vi "System_Host.vi"() -> ()   [LabVIEW 2017]
uses:
  <vilib>/Analysis/baseanly.llb/Mean (DBL).vi
  <vilib>/Utility/file.llb/Read Delimited Spreadsheet (string).vi
  <vilib>/Utility/file.llb/Write Delimited Spreadsheet (string).vi
  <vilib>/Utility/file.llb/Read Delimited Spreadsheet (DBL).vi
  <vilib>/Utility/file.llb/Write Delimited Spreadsheet (DBL).vi
  <resource>/objmgr/ni.dex.rc
  <vilib>/Analysis/NI_AALBase.lvlib
panel:
  in  "Flow Data?":bool=TRUE
  out "System Safe":bool
  in  "Exit Profile":bool
  in  "Select Operation Mode":T1(ring) caption="Select Operation Mode2"
  in  "CTAH Frequency\n[10*Hz]":u16
  out "System Time [s]":sgl
  out "System Loop Time (ms)":u32
  in  "Load Power Profile":bool
  in  "Dyn. Power Profile File":path
  out "CTAH Temperatures":T2(graph)
  out "CTAH Outlet":dbl format="%0.2f"
  out "CTAH Inlet":dbl format="%0.2f"
  out "Core Temperatures":T2(graph)
  out "Heater Outlet":dbl format="%0.2f"
  out "Heater Inlet":dbl format="%0.2f"
  out "Core Power":T2(graph)
  out "FM-60 [kg/s]":sgl
  out "FM-40 [kg/s]":sgl
  out "FM-30 [kg/s]":sgl
  out "FM-20 [kg/s]":sgl
  in  "Tab Control":enum32{"Thermocouple Readings [C]"}(tab)
  out "WT-10":sgl
  out "BT-11":sgl
  out "BT-12":sgl
  out "WT-13":sgl
  out "CX-10":dbl format="%0.2f"
  out "CX-11":dbl format="%0.2f"
  out "WT-20":sgl
  out "BT-21":sgl
  out "WT-22":sgl
  out "BT-23":sgl
  out "WT-24":sgl
  out "BT-25":sgl
  out "WT-26":sgl
  out "BT-27":sgl
  out "WT-28":sgl
  out "BT-29":sgl
  out "BT-30":sgl
  out "WT-31":sgl
  out "BT-32":sgl
  out "WT-33":sgl
  out "BT-34":sgl
  out "WT-35":sgl
  out "WT-40":sgl
  out "BT-41":sgl
  out "WT-42":sgl
  out "BT-43":sgl
  out "BT-60":sgl
  out "WT-61":sgl
  out "WT-62":sgl
  out "BT-63":sgl
  out "WT-64":sgl
  out "BT-65":sgl
  out "BT-66":sgl
  out "WT-67":sgl
  out "ST-10":sgl
  out "ST-11":sgl
  out "ST-12":sgl[](array[numeric])
  out "ST-13":sgl
  out "ST-14":sgl[](array[numeric])
  out "AT-01":sgl
  out "AT-02":sgl
  out "Profile Step":i32
  out "Power Output [W]":dbl
  out "Power Input Signal [W]":dbl
  out "Output Current 2 [A]":dbl
  out "Output Voltage 2 [V]":dbl
  out "Output Current 1 [A]":dbl
  out "Output Voltage 1 [V]":dbl
  out "Loop Period [ms]":i64
  in  "Shutdown":bool
  in  "Desired Power [W]":dbl
  in  "Power Output On":bool
  in  "Pump Frequency\n[10*Hz]":u16
  in  "ACTIVATE - PUMP":bool
  in  "Pump Operation Mode":i32(listbox)
  in  "TCHX Frequency\n[10*Hz]":u16
  in  "ACTIVATE - TCHX":bool
  in  "TCHX Operation Mode":i32(listbox)
  in  "VFD Stop":bool
  in  "ACTIVATE - CTAH":bool
  in  "CTAH Operation Mode":i32(listbox)
  in  "Error In":errorcluster
  out "Number of Disconnections":u32
  out "Available Elements for Reading":i32
  out "DAQ?":bool
  in  "Stop DAQ":bool
  out "Error Out":errorcluster
  # ".csv file with single column\nAssume constant loop frequency (1 Hz)"
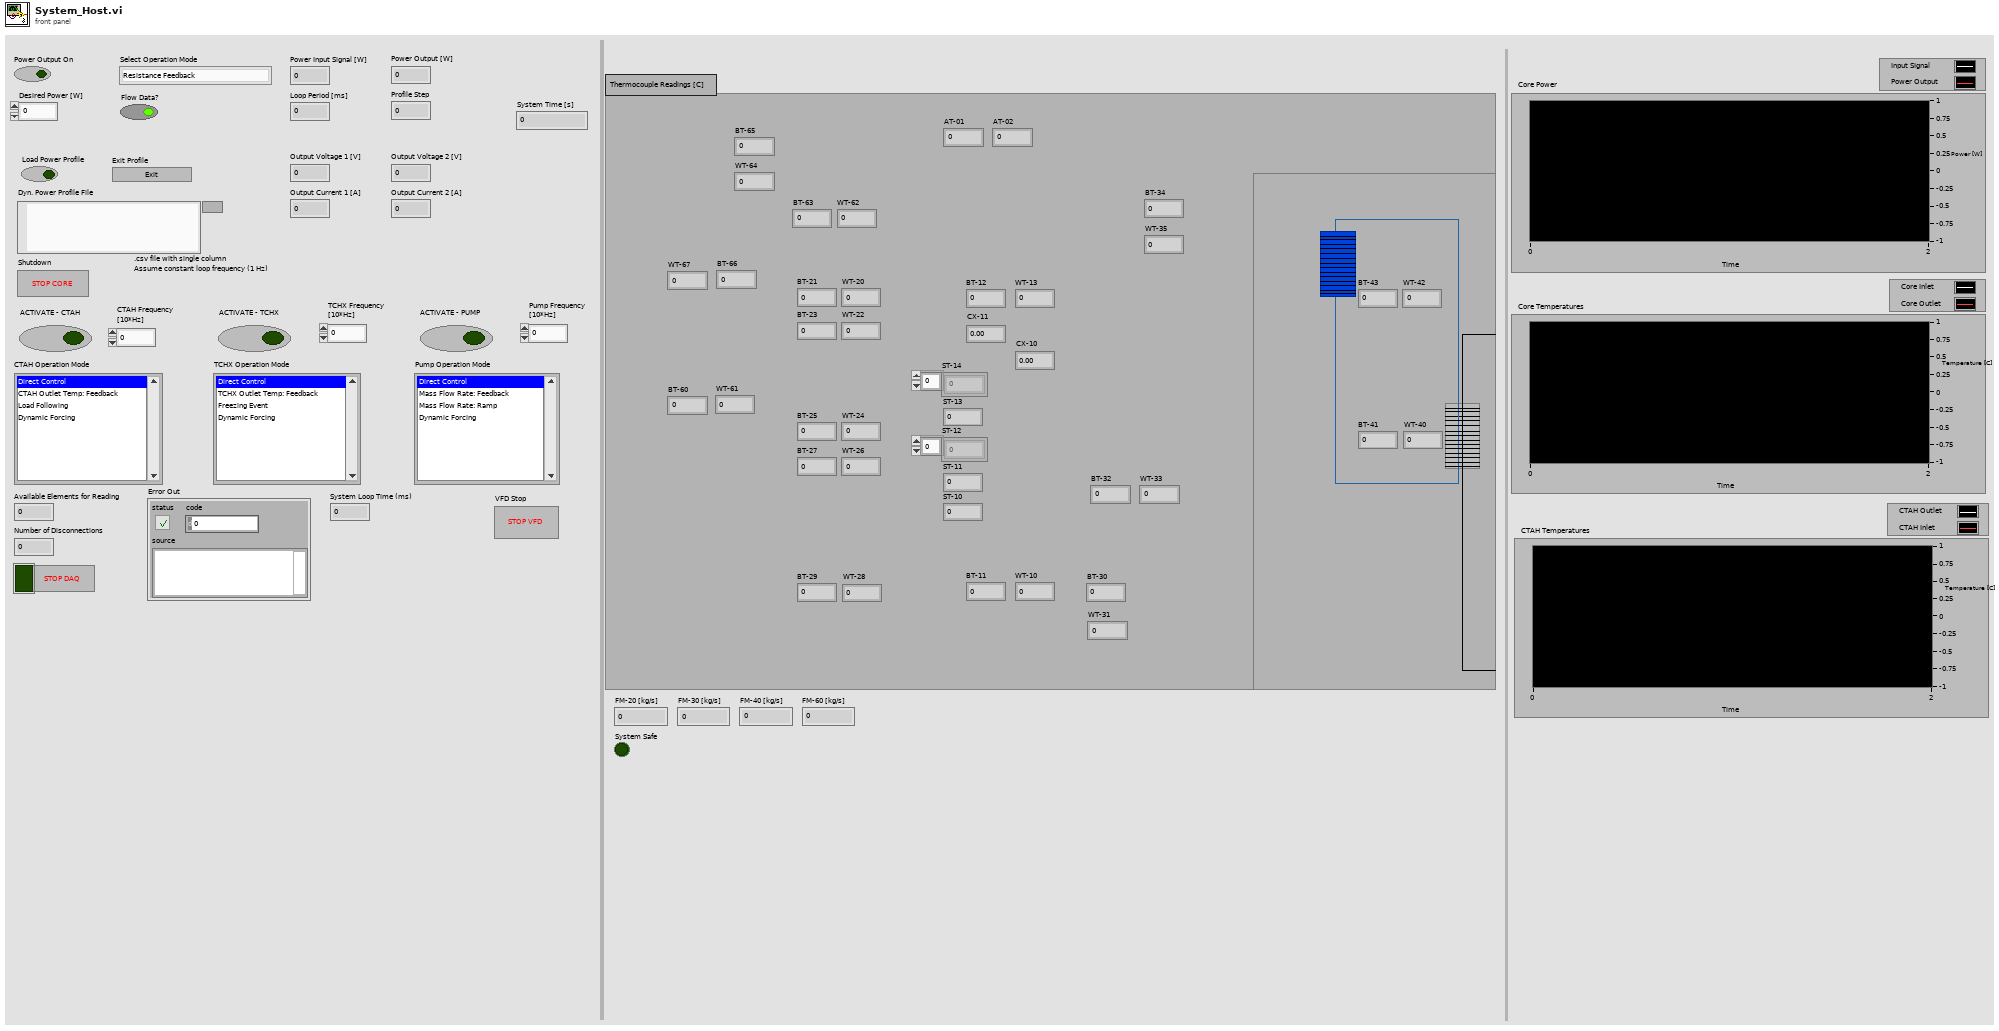
[diagram p1: front panel]
types:
  T1 = enum16{"Resistance Feedback", "Power Profile Input", "Resistance Feedback_Analog", "Power Profile Input_Analog", "SNF Digital", "SNF Analog\n", "Shutdown"}
  T2 = cluster{"Power Input Signal":dbl, "Power Output":dbl}
  T3 = cluster{"Power Input Signal [W]":dbl, "Power Output [W]":dbl}
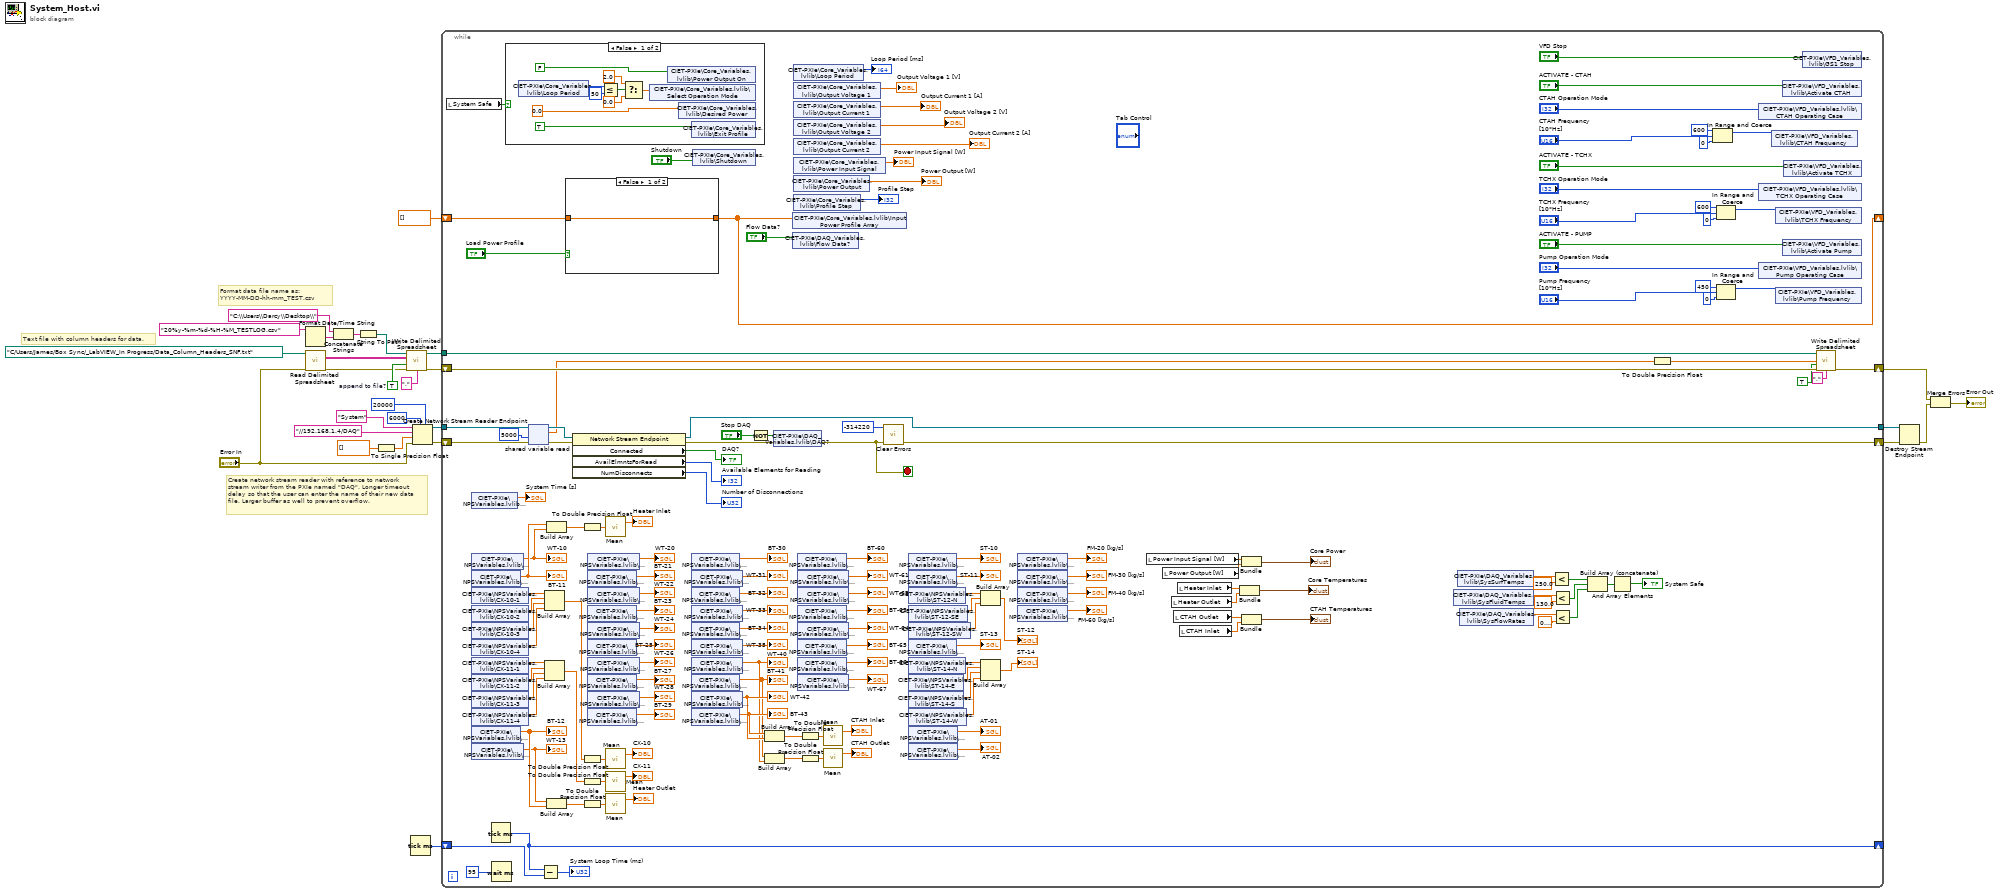
[diagram p0: block diagram]
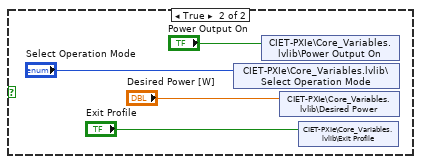
[diagram p2: hidden frame]
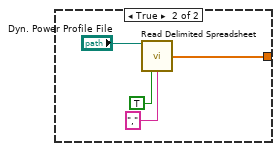
[diagram p3: hidden frame]
diagram:
  w15 = TRUE  # append to file?
  # "Format data file name as:\nYYYY-MM-DD-hh-mm_TEST.csv"
  # "Create network stream reader with reference to network\nstream writer from the PXIe named \"DAQ\". Longer timeout\ndelay so that the user can enter the name of their new data\nfile. Larger buffer as well to prevent overflow."
  # "Text file with column headers for data."
  n1 = Format Date/Time String(time format string (%c)="20%y-%m-%d-%H-%M_TESTLOG.csv") -> (date/time string=w5:string)  [unwired: 2 in]
  n2 = call-poly <vilib>:"Read Delimited Spreadsheet.vi"("file path (dialog if empty)"=path "C:/Users/James/Box Sync/_LabVIEW_In Progress/Data_Column_Headers_SNF.txt", "error in (no error)"="Error In") -> ("all rows"=w18:string[][], "error out"=w13:errorcluster)  [unwired: 8 in, 4 out]
  n3 = Concatenate Strings("C:\\Users\\Darcy\\Desktop\\" ("string"), w5) -> (w7:string)
  n4 = String To Path(string=w7) -> (path=w4:path)
  n5 = To Single Precision Float(number=dbl[] []) -> (single precision float=w26:sgl[])
  n6 = call-poly <vilib>:"Write Delimited Spreadsheet.vi"("file path (dialog if empty)"=w4, "2D data"=w18, "append to file? (new file:F)"=w15, "error in (no error)"=w13, "delimiter (\\t)"=",") -> ("new file path (Not A Path if cancelled)"=w14:path, "error out"=w12:errorcluster)  [unwired: 9 in]
  n7 = Tick Count (ms)() -> (millisecond timer value=w1:u32)
  n8 = Create Network Stream Reader Endpoint(5:20000 ("timeout in ms (-1)"), 7:6000 ("reader buffer size"), 8:"Error In", 9:w26, 10:"//192.168.1.4/DAQ" ("writer url"), 11:"System" ("reader name")) -> (0:w23:errorcluster, 3:w22:refnum<k21>)  [unwired: 1 in]
  n9 = while {
    shift-right: [w173] -> w21
    shift-left: w23 -> [w181]
    tunnel: w22 -> [w182]
    tunnel: [w172] -> w20
    tunnel: w14 -> [w168]
    shift-right: [w166] -> w11
    shift-left: w12 -> [w167]
    shift-right: [w52] -> _
    shift-left: dbl[] [] ("Input Power Profile Array") -> [w53]
    shift-right: [w49] -> _
    shift-left: w1 -> [w50]
    stop <- w171 stop-if-true
    n10 = local read "System Safe"() -> (w31:bool)
    n11 = shared-variable "CIET-PXIe\\NPSVariables.lvlib\\Time"() -> (→"System Time [s]":sgl)  [unwired: 1 in, 1 out]
    n12 = shared-variable "CIET-PXIe\\NPSVariables.lvlib\\WT-10"() -> (w73:sgl)  [unwired: 1 in, 1 out]
    "WT-10" <- w73
    n13 = shared-variable "CIET-PXIe\\NPSVariables.lvlib\\BT-11"() -> (w74:sgl)  [unwired: 1 in, 1 out]
    "BT-11" <- w74
    n14 = shared-variable "CIET-PXIe\\NPSVariables.lvlib\\CX-10-1"() -> (w139:sgl)  [unwired: 1 in, 1 out]
    n15 = shared-variable "CIET-PXIe\\NPSVariables.lvlib\\CX-10-2"() -> (w138:sgl)  [unwired: 1 in, 1 out]
    n16 = shared-variable "CIET-PXIe\\NPSVariables.lvlib\\CX-10-3"() -> (w137:sgl)  [unwired: 1 in, 1 out]
    n17 = shared-variable "CIET-PXIe\\NPSVariables.lvlib\\CX-10-4"() -> (w136:sgl)  [unwired: 1 in, 1 out]
    n18 = shared-variable "CIET-PXIe\\NPSVariables.lvlib\\CX-11-1"() -> (w132:sgl)  [unwired: 1 in, 1 out]
    n19 = shared-variable "CIET-PXIe\\NPSVariables.lvlib\\CX-11-2"() -> (w131:sgl)  [unwired: 1 in, 1 out]
    n20 = shared-variable "CIET-PXIe\\NPSVariables.lvlib\\CX-11-3"() -> (w130:sgl)  [unwired: 1 in, 1 out]
    n21 = shared-variable "CIET-PXIe\\NPSVariables.lvlib\\CX-11-4"() -> (w129:sgl)  [unwired: 1 in, 1 out]
    n22 = shared-variable "CIET-PXIe\\NPSVariables.lvlib\\BT-12"() -> (w78:sgl)  [unwired: 1 in, 1 out]
    "BT-12" <- w78
    n23 = shared-variable "CIET-PXIe\\NPSVariables.lvlib\\WT-13"() -> (w77:sgl)  [unwired: 1 in, 1 out]
    "WT-13" <- w77
    n24 = Tick Count (ms)() -> (millisecond timer value=w49:u32)
    n25 = Wait (ms)(milliseconds to wait=u32 95) -> ()  [unwired: 1 out]
    n26 = case shown="False" w31 {
      frame False {
        n27 = shared-variable "CIET-PXIe\\Core_Variables.lvlib\\Loop Period"() -> (w189:i64)  [unwired: 1 in, 1 out]
        n28 = Less Or Equal?(x=w189, y=i64 50) -> (x <= y?=w190:bool)
        n29 = Select(t=2.0, s=w190, f=0.0) -> (s? t:f=w185:dbl)
        n30 = shared-variable "CIET-PXIe\\Core_Variables.lvlib\\Select Operation Mode"(w185) -> ()  [unwired: 1 in, 1 out]
        n31 = shared-variable "CIET-PXIe\\Core_Variables.lvlib\\Power Output On"(FALSE ("Power Output On")) -> ()  [unwired: 1 in, 1 out]
        n32 = shared-variable "CIET-PXIe\\Core_Variables.lvlib\\Desired Power"(0.0 ("Desired Power")) -> ()  [unwired: 1 in, 1 out]
        n33 = shared-variable "CIET-PXIe\\Core_Variables.lvlib\\Exit Profile"(TRUE ("Exit Profile")) -> ()  [unwired: 1 in, 1 out]
      }
      frame True {
        n34 = shared-variable "CIET-PXIe\\Core_Variables.lvlib\\Select Operation Mode"("Select Operation Mode") -> ()  [unwired: 1 in, 1 out]
        n35 = shared-variable "CIET-PXIe\\Core_Variables.lvlib\\Power Output On"("Power Output On") -> ()  [unwired: 1 in, 1 out]
        n36 = shared-variable "CIET-PXIe\\Core_Variables.lvlib\\Desired Power"("Desired Power [W]") -> ()  [unwired: 1 in, 1 out]
        n37 = shared-variable "CIET-PXIe\\Core_Variables.lvlib\\Exit Profile"("Exit Profile") -> ()  [unwired: 1 in, 1 out]
      }
    }
    n38 = shared-variable-read(w182, w181, 5000 ("timeout ms (-1)")) -> (w178:refnum<k21>, w176:errorcluster, w140:sgl[])  [unwired: 1 out]
    n39 = Subtract(x=w49, y=w50) -> (x-y=→"System Loop Time (ms)":u32)
    n40 = Build Array(w139, w138, w137, w136) -> (w135:sgl[])
    n41 = Build Array(w132, w131, w130, w129) -> (w128:sgl[])
    n42 = Build Array(w74, w73) -> (w75:sgl[])
    n43 = Build Array(w77, w78) -> (w79:sgl[])
    n44 = case shown="False" "Load Power Profile" {
      tunnel: [w198 w199] -> w52
      tunnel: w53 -> [w198 _]
      frame False {
      }
      frame True {
        n45 = call-poly <vilib>:"Read Delimited Spreadsheet.vi"("file path (dialog if empty)"="Dyn. Power Profile File", "transpose? (F)"=TRUE, "delimiter (\\t)"="," ("delimiter (\\t)")) -> ("first row"=w199:dbl[])  [unwired: 7 in, 5 out]
      }
    }
    n46 = property class="Network Stream Endpoint"(reference=w178, error in=w176) -> (reference out=w172:refnum<k21>, error out=w177:errorcluster, "Connected"=→"DAQ?":bool, "AvailElmntsForRead"=→"Available Elements for Reading":i32, "NumDisconnects"=→"Number of Disconnections":u32)
    n47 = To Double Precision Float(number=w75) -> (double precision float=w76:dbl[])
    n48 = To Double Precision Float(number=w135) -> (double precision float=w134:dbl[])
    n49 = To Double Precision Float(number=w128) -> (double precision float=w133:dbl[])
    n50 = To Double Precision Float(number=w79) -> (double precision float=w80:dbl[])
    n51 = shared-variable "CIET-PXIe\\NPSVariables.lvlib\\WT-20"() -> (→"WT-20":sgl)  [unwired: 1 in, 1 out]
    n52 = shared-variable "CIET-PXIe\\NPSVariables.lvlib\\BT-21"() -> (→"BT-21":sgl)  [unwired: 1 in, 1 out]
    n53 = shared-variable "CIET-PXIe\\NPSVariables.lvlib\\WT-22"() -> (→"WT-22":sgl)  [unwired: 1 in, 1 out]
    n54 = shared-variable "CIET-PXIe\\NPSVariables.lvlib\\BT-23"() -> (→"BT-23":sgl)  [unwired: 1 in, 1 out]
    n55 = shared-variable "CIET-PXIe\\NPSVariables.lvlib\\WT-24"() -> (→"WT-24":sgl)  [unwired: 1 in, 1 out]
    n56 = shared-variable "CIET-PXIe\\NPSVariables.lvlib\\BT-25"() -> (→"BT-25":sgl)  [unwired: 1 in, 1 out]
    n57 = shared-variable "CIET-PXIe\\NPSVariables.lvlib\\WT-26"() -> (→"WT-26":sgl)  [unwired: 1 in, 1 out]
    n58 = shared-variable "CIET-PXIe\\NPSVariables.lvlib\\BT-27"() -> (→"BT-27":sgl)  [unwired: 1 in, 1 out]
    n59 = shared-variable "CIET-PXIe\\NPSVariables.lvlib\\WT-28"() -> (→"WT-28":sgl)  [unwired: 1 in, 1 out]
    n60 = shared-variable "CIET-PXIe\\NPSVariables.lvlib\\BT-29"() -> (→"BT-29":sgl)  [unwired: 1 in, 1 out]
    n61 = call-poly <vilib>:"Mean.vi"("X"=w76) -> ("mean"=→"Heater Inlet":dbl)  [unwired: 1 out]
    n62 = call-poly <vilib>:"Mean.vi"("X"=w134) -> ("mean"=→"CX-10":dbl)  [unwired: 1 out]
    n63 = call-poly <vilib>:"Mean.vi"("X"=w133) -> ("mean"=→"CX-11":dbl)  [unwired: 1 out]
    n64 = call-poly <vilib>:"Mean.vi"("X"=w80) -> ("mean"=→"Heater Outlet":dbl)  [unwired: 1 out]
    n65 = shared-variable "CIET-PXIe\\NPSVariables.lvlib\\BT-30"() -> (→"BT-30":sgl)  [unwired: 1 in, 1 out]
    n66 = shared-variable "CIET-PXIe\\NPSVariables.lvlib\\WT-31"() -> (→"WT-31":sgl)  [unwired: 1 in, 1 out]
    n67 = shared-variable "CIET-PXIe\\NPSVariables.lvlib\\BT-32"() -> (→"BT-32":sgl)  [unwired: 1 in, 1 out]
    n68 = shared-variable "CIET-PXIe\\NPSVariables.lvlib\\WT-33"() -> (→"WT-33":sgl)  [unwired: 1 in, 1 out]
    n69 = shared-variable "CIET-PXIe\\NPSVariables.lvlib\\BT-34"() -> (→"BT-34":sgl)  [unwired: 1 in, 1 out]
    n70 = shared-variable "CIET-PXIe\\NPSVariables.lvlib\\WT-35"() -> (→"WT-35":sgl)  [unwired: 1 in, 1 out]
    n71 = shared-variable "CIET-PXIe\\NPSVariables.lvlib\\WT-40"() -> (w59:sgl)  [unwired: 1 in, 1 out]
    "WT-40" <- w59
    n72 = shared-variable "CIET-PXIe\\NPSVariables.lvlib\\BT-41"() -> (w58:sgl)  [unwired: 1 in, 1 out]
    "BT-41" <- w58
    n73 = shared-variable "CIET-PXIe\\NPSVariables.lvlib\\WT-42"() -> (w61:sgl)  [unwired: 1 in, 1 out]
    "WT-42" <- w61
    n74 = shared-variable "CIET-PXIe\\NPSVariables.lvlib\\BT-43"() -> (w60:sgl)  [unwired: 1 in, 1 out]
    "BT-43" <- w60
    n75 = shared-variable "CIET-PXIe\\Core_Variables.lvlib\\Shutdown"("Shutdown") -> ()  [unwired: 1 in, 1 out]
    n76 = Not(x="Stop DAQ") -> (.not. x?=w180:bool)
    n77 = Build Array(w60, w61) -> (w66:sgl[])
    n78 = Build Array(w58, w59) -> (w63:sgl[])
    n79 = shared-variable "CIET-PXIe\\DAQ_Variables.lvlib\\DAQ?"(w180, error in=w177) -> (error out=w171:errorcluster)
    n80 = shared-variable "CIET-PXIe\\Core_Variables.lvlib\\Input Power Profile Array"(w52) -> ()  [unwired: 1 in, 1 out]
    n81 = shared-variable "CIET-PXIe\\DAQ_Variables.lvlib\\Flow Data?"("Flow Data?") -> ()  [unwired: 1 in, 1 out]
    n82 = shared-variable "CIET-PXIe\\Core_Variables.lvlib\\Loop Period"() -> (→"Loop Period [ms]":i64)  [unwired: 1 in, 1 out]
    n83 = shared-variable "CIET-PXIe\\Core_Variables.lvlib\\Output Voltage 1"() -> (→"Output Voltage 1 [V]":dbl)  [unwired: 1 in, 1 out]
    n84 = shared-variable "CIET-PXIe\\Core_Variables.lvlib\\Output Current 1"() -> (→"Output Current 1 [A]":dbl)  [unwired: 1 in, 1 out]
    n85 = shared-variable "CIET-PXIe\\Core_Variables.lvlib\\Output Voltage 2"() -> (→"Output Voltage 2 [V]":dbl)  [unwired: 1 in, 1 out]
    n86 = shared-variable "CIET-PXIe\\Core_Variables.lvlib\\Output Current 2"() -> (→"Output Current 2 [A]":dbl)  [unwired: 1 in, 1 out]
    n87 = shared-variable "CIET-PXIe\\Core_Variables.lvlib\\Power Input Signal"() -> (→"Power Input Signal [W]":dbl)  [unwired: 1 in, 1 out]
    n88 = shared-variable "CIET-PXIe\\Core_Variables.lvlib\\Power Output"() -> (→"Power Output [W]":dbl)  [unwired: 1 in, 1 out]
    n89 = shared-variable "CIET-PXIe\\Core_Variables.lvlib\\Profile Step"() -> (→"Profile Step":i32)  [unwired: 1 in, 1 out]
    n90 = shared-variable "CIET-PXIe\\NPSVariables.lvlib\\BT-60"() -> (→"BT-60":sgl)  [unwired: 1 in, 1 out]
    n91 = shared-variable "CIET-PXIe\\NPSVariables.lvlib\\WT-61"() -> (→"WT-61":sgl)  [unwired: 1 in, 1 out]
    n92 = shared-variable "CIET-PXIe\\NPSVariables.lvlib\\WT-62"() -> (→"WT-62":sgl)  [unwired: 1 in, 1 out]
    n93 = shared-variable "CIET-PXIe\\NPSVariables.lvlib\\BT-63"() -> (→"BT-63":sgl)  [unwired: 1 in, 1 out]
    n94 = shared-variable "CIET-PXIe\\NPSVariables.lvlib\\WT-64"() -> (→"WT-64":sgl)  [unwired: 1 in, 1 out]
    n95 = shared-variable "CIET-PXIe\\NPSVariables.lvlib\\BT-65"() -> (→"BT-65":sgl)  [unwired: 1 in, 1 out]
    n96 = shared-variable "CIET-PXIe\\NPSVariables.lvlib\\BT-66"() -> (→"BT-66":sgl)  [unwired: 1 in, 1 out]
    n97 = shared-variable "CIET-PXIe\\NPSVariables.lvlib\\WT-67"() -> (→"WT-67":sgl)  [unwired: 1 in, 1 out]
    n98 = To Double Precision Float(number=w66) -> (double precision float=w67:dbl[])
    n99 = To Double Precision Float(number=w63) -> (double precision float=w64:dbl[])
    n100 = call-poly <vilib>:"Mean.vi"("X"=w67) -> ("mean"=→"CTAH Inlet":dbl)  [unwired: 1 out]
    n101 = call-poly <vilib>:"Mean.vi"("X"=w64) -> ("mean"=→"CTAH Outlet":dbl)  [unwired: 1 out]
    n102 = call <vilib>:"Clear Errors.vi"("error in (no error)"=w171, "specific error code to clear (0: all)"=-314220) -> ("error out"=w173:errorcluster)  [unwired: 4 in, 1 out]
    n103 = shared-variable "CIET-PXIe\\NPSVariables.lvlib\\ST-10"() -> (→"ST-10":sgl)  [unwired: 1 in, 1 out]
    n104 = shared-variable "CIET-PXIe\\NPSVariables.lvlib\\ST-11"() -> (→"ST-11":sgl)  [unwired: 1 in, 1 out]
    n105 = shared-variable "CIET-PXIe\\NPSVariables.lvlib\\ST-12-N"() -> (w99:sgl)  [unwired: 1 in, 1 out]
    n106 = shared-variable "CIET-PXIe\\NPSVariables.lvlib\\ST-12-SE"() -> (w98:sgl)  [unwired: 1 in, 1 out]
    n107 = shared-variable "CIET-PXIe\\NPSVariables.lvlib\\ST-12-SW"() -> (w97:sgl)  [unwired: 1 in, 1 out]
    n108 = shared-variable "CIET-PXIe\\NPSVariables.lvlib\\ST-13"() -> (→"ST-13":sgl)  [unwired: 1 in, 1 out]
    n109 = shared-variable "CIET-PXIe\\NPSVariables.lvlib\\ST-14-N"() -> (w94:sgl)  [unwired: 1 in, 1 out]
    n110 = shared-variable "CIET-PXIe\\NPSVariables.lvlib\\ST-14-E"() -> (w93:sgl)  [unwired: 1 in, 1 out]
    n111 = shared-variable "CIET-PXIe\\NPSVariables.lvlib\\ST-14-S"() -> (w92:sgl)  [unwired: 1 in, 1 out]
    n112 = shared-variable "CIET-PXIe\\NPSVariables.lvlib\\ST-14-W"() -> (w91:sgl)  [unwired: 1 in, 1 out]
    n113 = shared-variable "CIET-PXIe\\NPSVariables.lvlib\\AT-01"() -> (→"AT-01":sgl)  [unwired: 1 in, 1 out]
    n114 = shared-variable "CIET-PXIe\\NPSVariables.lvlib\\AT-02"() -> (→"AT-02":sgl)  [unwired: 1 in, 1 out]
    n115 = Build Array(w99, w98, w97) -> (→"ST-12":sgl[])
    n116 = Build Array(w94, w93, w92, w91) -> (→"ST-14":sgl[])
    n117 = shared-variable "CIET-PXIe\\NPSVariables.lvlib\\FM-20"() -> (→"FM-20 [kg/s]":sgl)  [unwired: 1 in, 1 out]
    n118 = shared-variable "CIET-PXIe\\NPSVariables.lvlib\\FM-30"() -> (→"FM-30 [kg/s]":sgl)  [unwired: 1 in, 1 out]
    n119 = shared-variable "CIET-PXIe\\NPSVariables.lvlib\\FM-40"() -> (→"FM-40 [kg/s]":sgl)  [unwired: 1 in, 1 out]
    n120 = shared-variable "CIET-PXIe\\NPSVariables.lvlib\\FM-60"() -> (→"FM-60 [kg/s]":sgl)  [unwired: 1 in, 1 out]
    n121 = local read "Power Input Signal [W]"() -> (w83:dbl)
    n122 = local read "Power Output [W]"() -> (w82:dbl)
    n123 = local read "Heater Outlet"() -> (w68:dbl)
    n124 = local read "CTAH Outlet"() -> (w56:dbl)
    n125 = local read "Heater Inlet"() -> (w69:dbl)
    n126 = local read "CTAH Inlet"() -> (w55:dbl)
    n127 = Bundle("Heater Inlet"=w69, "Heater Outlet"=w68) -> (→"Core Temperatures":cluster{"Heater Inlet":dbl, "Heater Outlet":dbl})  [unwired: 1 in]
    n128 = Bundle("Power Input Signal [W]"=w83, "Power Output [W]"=w82) -> (→"Core Power":T3)  [unwired: 1 in]
    n129 = Bundle("CTAH Outlet"=w56, "CTAH Inlet"=w55) -> (→"CTAH Temperatures":cluster{"CTAH Outlet":dbl, "CTAH Inlet":dbl})  [unwired: 1 in]
    n130 = shared-variable "CIET-PXIe\\DAQ_Variables.lvlib\\SysFluidTemps"() -> (w37:sgl[])  [unwired: 1 in, 1 out]
    n131 = shared-variable "CIET-PXIe\\DAQ_Variables.lvlib\\SysSurfTemps"() -> (w39:sgl[])  [unwired: 1 in, 1 out]
    n132 = shared-variable "CIET-PXIe\\DAQ_Variables.lvlib\\SysFlowRates"() -> (w35:sgl[])  [unwired: 1 in, 1 out]
    n133 = Less?(x=w39, y=sgl 250.0) -> (x < y?=w41:bool[])
    n134 = Less?(x=w37, y=sgl 130.0) -> (x < y?=w34:bool[])
    n135 = Less?(x=w35, y=sgl 0.2) -> (x < y?=w33:bool[])
    n136 = Build Array (concatenate)(w41, w34, w33) -> (w42:bool[])
    n137 = And Array Elements(Boolean array=w42) -> (logical AND=→"System Safe":bool)
    n138 = To Double Precision Float(number=w140) -> (double precision float=w51:dbl[])
    n139 = In Range and Coerce(upper limit=u16 600, x="CTAH Frequency\n[10*Hz]", lower limit=u16 0) -> (coerced(x)=w46:u16)  [unwired: 1 out]
    n140 = In Range and Coerce(upper limit=u16 600, x="TCHX Frequency\n[10*Hz]", lower limit=u16 0) -> (coerced(x)=w158:u16)  [unwired: 1 out]
    n141 = In Range and Coerce(upper limit=u16 450, x="Pump Frequency\n[10*Hz]", lower limit=u16 0) -> (coerced(x)=w152:u16)  [unwired: 1 out]
    n142 = shared-variable "CIET-PXIe\\VFD_Variables.lvlib\\CTAH Operating Case"("CTAH Operation Mode") -> ()  [unwired: 1 in, 1 out]
    n143 = shared-variable "CIET-PXIe\\VFD_Variables.lvlib\\Pump Operating Case"("Pump Operation Mode") -> ()  [unwired: 1 in, 1 out]
    n144 = shared-variable "CIET-PXIe\\VFD_Variables.lvlib\\TCHX Operating Case"("TCHX Operation Mode") -> ()  [unwired: 1 in, 1 out]
    n145 = shared-variable "CIET-PXIe\\VFD_Variables.lvlib\\CTAH Frequency"(w46) -> ()  [unwired: 1 in, 1 out]
    n146 = shared-variable "CIET-PXIe\\VFD_Variables.lvlib\\Pump Frequency"(w152) -> ()  [unwired: 1 in, 1 out]
    n147 = shared-variable "CIET-PXIe\\VFD_Variables.lvlib\\TCHX Frequency"(w158) -> ()  [unwired: 1 in, 1 out]
    n148 = shared-variable "CIET-PXIe\\VFD_Variables.lvlib\\Activate CTAH"("ACTIVATE - CTAH") -> ()  [unwired: 1 in, 1 out]
    n149 = shared-variable "CIET-PXIe\\VFD_Variables.lvlib\\Activate Pump"("ACTIVATE - PUMP") -> ()  [unwired: 1 in, 1 out]
    n150 = shared-variable "CIET-PXIe\\VFD_Variables.lvlib\\Activate TCHX"("ACTIVATE - TCHX") -> ()  [unwired: 1 in, 1 out]
    n151 = shared-variable "CIET-PXIe\\VFD_Variables.lvlib\\GS1 Stop"("VFD Stop") -> ()  [unwired: 1 in, 1 out]
    n152 = call-poly <vilib>:"Write Delimited Spreadsheet.vi"("file path (dialog if empty)"=w168, "1D data"=w51, "append to file? (new file:F)"=TRUE, "error in (no error)"=w167, "delimiter (\\t)"="," ("delimiter (\\t)")) -> ("error out"=w166:errorcluster)  [unwired: 9 in, 1 out]
  }
  n153 = Destroy Stream Endpoint(8:w21, 11:w20) -> (0:w10:errorcluster)
  n154 = Merge Errors(w11, w10) -> (→"Error Out":errorcluster)
